vi "IPS120_GoToField.vi"(8 "error in":errorcluster, 10 "put into persistent mode after reaching target field?":bool, 11 "IPS120 Targets":T1={"Target Field (T)"=0.1, "Target Field Rate (T/min)"=0.1} {"Target Field (T)" format="%.4g"; "Target Field Rate (T/min)" format="%.4g"}) -> (0 "error out":errorcluster)   [LabVIEW 2016, in "IPS-120-API.lvlib"]
doc: "Use this VI to remotely interact with the Oxford Mercury power supply through \"Oxford-1820-Main.vi\", which MUST also be running."
uses:
  IPS-120-API.lvlib
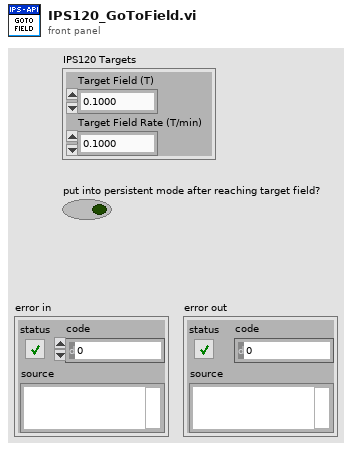
[diagram p1: front panel]
types:
  T1 = cluster{"Target Field (T)":dbl, "Target Field Rate (T/min)":dbl}
  T2 = cluster{"Magnet Field":dbl, "PS Field":dbl, "Target Field":dbl, "Target Field Rate":dbl, "Voltage":dbl, "Current":dbl, "Switch":bool}
  T3 = cluster{"Hold":bool, "Clamp":bool, "To Set":bool, "To Zero":bool, "Send to IPS":bool, "PS Heat":bool}
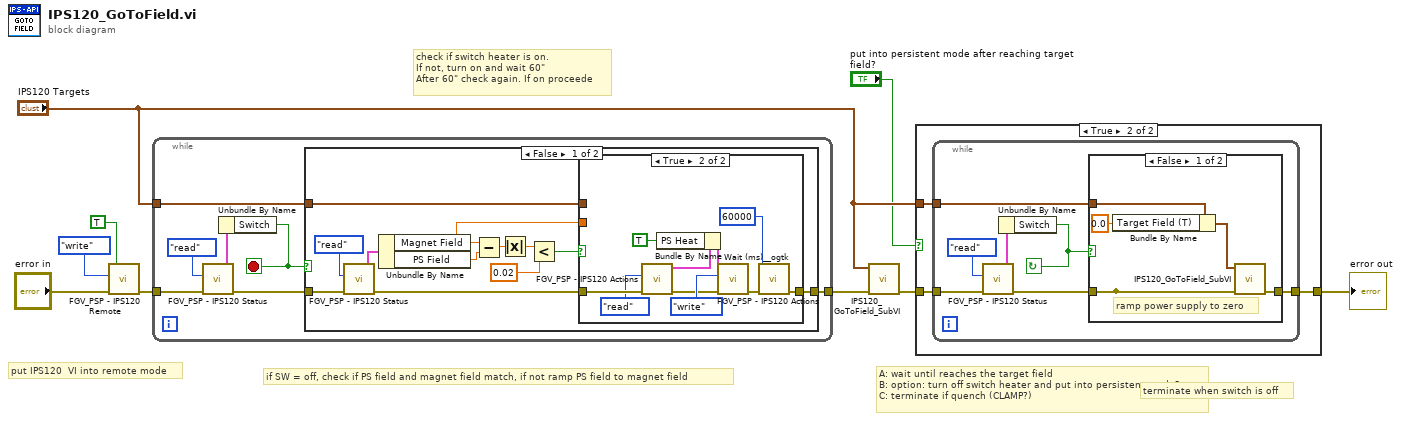
[diagram p0: block diagram]
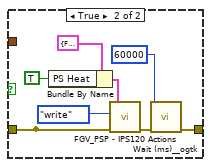
[diagram p3: hidden frame]
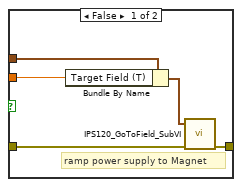
[diagram p4: hidden frame]
diagram:
  # "terminate when switch is off"
  # "A: wait until reaches the target field\nB: option: turn off switch heater and put into persistent mode?\nC: terminate if quench (CLAMP?)"
  # "if SW = off, check if PS field and magnet field match, if not ramp PS field to magnet field"
  # "check if switch heater is on.\nIf not, turn on and wait 60\"\nAfter 60\" check again. If on proceede"
  # "put IPS120  VI into remote mode"
  n1 = call "FGV_PSP - IPS120 Remote.vi"("error in"="error in", "Function"=enum16{"write", "read"}."write", "Remote"=TRUE ("Mercury Remote")) -> ("error out"=w8:errorcluster)  [unwired: 3 in, 1 out]
  n2 = while {
    tunnel: [w13] -> w9
    tunnel: w8 -> [w12]
    tunnel: "IPS120 Targets" -> [w10]
    stop <- w14 stop-if-true
    n3 = call "FGV_PSP - IPS120 Status.vi"("error in"=w12, "Function"=enum16{"write", "read"}."read") -> ("error out"=w15:errorcluster, "status"=w16:T2)  [unwired: 4 in]
    n4 = Unbundle By Name(w16) -> ("Switch"=w14:bool)
    n5 = case shown="False" w14 {
      tunnel: w15 -> [w27 w44]
      tunnel: [w28 w44] -> w13
      tunnel: w10 -> [w19 _]
      frame False {
        n6 = call "FGV_PSP - IPS120 Status.vi"("error in"=w27, "Function"=enum16{"write", "read"}."read") -> ("error out"=w25:errorcluster, "status"=w26:T2)  [unwired: 4 in]
        n7 = Unbundle By Name(w26) -> ("Magnet Field"=w18:dbl, "PS Field"=w24:dbl)
        n8 = Subtract(x=w18, y=w24) -> (x-y=w23:dbl)
        n9 = Absolute Value(x=w23) -> (abs(x)=w22:dbl)
        n10 = Less?(x=w22, y=0.02) -> (x < y?=w20:bool)
        n11 = case shown="True" w20 {
          tunnel: [w32 w40] -> w28
          tunnel: w25 -> [w33 w38]
          tunnel: w19 -> [w31 _]
          tunnel: w18 -> [w30 _]
          frame False {
            # "ramp power supply to Magnet"
            n12 = Bundle By Name(cluster=w31, "Target Field (T)"=w30) -> (w29:T1)
            n13 = call "IPS120_GoToField_SubVI.vi"("error in (no error)"=w33, "Mercury Targets"=w29) -> ("error out"=w32:errorcluster)  [unwired: 9 in]
          }
          frame True {
            n14 = call "FGV_PSP - IPS120 Actions.vi"("error in"=w38, "Function"=enum16{"write", "read"}."read") -> ("error out"=w37:errorcluster, "actions"=w36:T3)  [unwired: 4 in]
            n15 = Bundle By Name(cluster=w36, "PS Heat"=TRUE ("Send to IPS")) -> (w35:T3)
            n16 = call "FGV_PSP - IPS120 Actions.vi"("error in"=w37, "Function"=enum16{"write", "read"}."write", "actions"=w35) -> ("error out"=w41:errorcluster)  [unwired: 3 in, 1 out]
            n17 = call <userlib>:"Wait (ms)__ogtk.vi"("error in (no error)"=w41, "milliseconds to wait"=u32 60000) -> ("error out"=w40:errorcluster)  [unwired: 8 in, 1 out]
          }
        }
      }
      frame True {
      }
    }
  }
  n18 = call "IPS120_GoToField_SubVI.vi"("error in (no error)"=w9, "Mercury Targets"="IPS120 Targets") -> ("error out"=w4:errorcluster)  [unwired: 9 in]
  n19 = case shown="True" "put into persistent mode after reaching target field?" {
    tunnel: w4 -> [w45 w48]
    tunnel: "IPS120 Targets" -> [_ w47]
    tunnel: [w45 w46] -> w2
    frame False {
    }
    frame True {
      n20 = while {
        tunnel: [w54] -> w46
        tunnel: w48 -> [w53]
        tunnel: w47 -> [w51]
        stop <- w49 continue-if-true
        n21 = call "FGV_PSP - IPS120 Status.vi"("error in"=w53, "Function"=enum16{"write", "read"}."read") -> ("error out"=w50:errorcluster, "status"=w55:T2)  [unwired: 4 in]
        n22 = Unbundle By Name(w55) -> ("Switch"=w49:bool)
        n23 = case shown="False" w49 {
          tunnel: [w60 w63] -> w54
          tunnel: [w56 w61] -> _
          tunnel: w51 -> [w59 _]
          tunnel: w50 -> [w56 w61]
          frame False {
            # "ramp power supply to zero"
            n24 = Bundle By Name(cluster=w59, "Target Field (T)"=0.0) -> (w58:T1)
            n25 = call "IPS120_GoToField_SubVI.vi"("error in (no error)"=w56, "Mercury Targets"=w58) -> ("error out"=w60:errorcluster)  [unwired: 9 in]
          }
          frame True {
            n26 = Bundle By Name(cluster=T3 {"Hold"=FALSE, "Clamp"=FALSE, "To Set"=FALSE, "To Zero"=FALSE, "Send to IPS"=FALSE, "PS Heat"=FALSE} ("mercury actions"), "PS Heat"=TRUE ("Send to IPS")) -> (w65:T3)
            n27 = call "FGV_PSP - IPS120 Actions.vi"("error in"=w61, "Function"=enum16{"write", "read"}."write", "actions"=w65) -> ("error out"=w64:errorcluster)  [unwired: 3 in, 1 out]
            n28 = call <userlib>:"Wait (ms)__ogtk.vi"("error in (no error)"=w64, "milliseconds to wait"=u32 60000) -> ("error out"=w63:errorcluster)  [unwired: 8 in, 1 out]
          }
        }
      }
    }
  }
  "error out" <- w2
